vi "MegaVIEW_v_0_0_0.vi"() -> ()   [LabVIEW 2016]
panel:
  in  "Tab Control":enum32{"Setup", "Measure"}(tab)
  in  "Initalize Tempmonitor":bool
  in  "Initalize Multimeter":bool
  in  "Initalize Gaussmeter 3":bool
  in  "Initalize Gaussmeter 2":bool
  in  "Initalize Gaussmeter 1":bool
  in  "Mobile Sensor":enum32{"Sensor 1", "Sensor 2", "Sensor 3"}(radio)
  in  "Multimeter":bool
  in  "Gaussmeter 1":bool
  in  "Gaussmeter 2":bool
  in  "Gaussmeter 3":bool
  in  "Tempmonitor":bool
  in  "VISA Gaussmeter 1":refnum<visa-resource-name>
  in  "VISA Gaussmeter 2":refnum<visa-resource-name>
  in  "VISA Gaussmeter 3":refnum<visa-resource-name>
  in  "VISA Multimeter":refnum<visa-resource-name>
  in  "VISA Tempmonitor":refnum<visa-resource-name>
  in  "Method":u16(ring) items=["50 A - 50 mV Shunt", "Direct: 3 A Mode, front", "Direct: 3 A Mode, rear", "Direct: 10 A Mode"]
  in  "Type 1":u16(ring) items=["Reference (current replacement)", "Main", "Main: x-component", "Main: y-component", "Main: z-component"]
  in  "Type 2":u16(ring)
  in  "Type 3":u16(ring)
  in  "x1 [mm]":dbl
  in  "y1 [mm]":dbl
  in  "z1 [mm]":dbl
  in  "x2 [mm]":dbl
  in  "y2 [mm]":dbl
  in  "z2 [mm]":dbl
  in  "x3 [mm]":dbl
  in  "y3 [mm]":dbl
  in  "z3 [mm]":dbl
  in  "Zero Sensor 1":bool
  in  "Zero Sensor 2":bool
  in  "Zero Sensor 3":bool
  in  "Measurement Rate [Hz]":dbl
  in  "Duration [s]":dbl
  in  "Current\nReedings":dbl
  in  "Field\nReadings":dbl
  in  "Randomize Positions":bool
  in  "Position File":path
  in  "Mode":bool
  in  "hours":dbl
  in  "seconds":dbl
  in  "minutes":dbl
  in  "exit":bool
  in  "Main Graph: y-axis":u16(ring) items=["B int [mT]", "B ref [mT]", "B1 [mT]", "B2 [mT]", "B3 [mT]", "T [K]", ""]
  out "Output File":path
  out "t [s]":dbl
  out "x [mm]":dbl
  out "y [mm]":dbl
  out "z [mm]":dbl
  out "I [A]":dbl
  out "B1 [mT]":dbl
  out "B2 [mT]":dbl
  out "B3 [mT]":dbl
  out "T [K]":dbl
  in  "stop":bool
  in  "start":bool
  out "Field 1 Graph":cluster{"X":dbl, "Y":dbl}[](graph)
  out "Current Graph":cluster{"X":dbl, "Y":dbl}[](graph)
  out "Temperature Graph":cluster{"X":dbl, "Y":dbl}[](graph)
  out "Field 2 Graph":cluster{"X":dbl, "Y":dbl}[](graph)
  out "Field 3 Graph":cluster{"X":dbl, "Y":dbl}[](graph)
  out "Main Graph":cluster{"X":dbl, "Y":dbl}[](graph)
  in  "Main Graph: x-axis":u16(ring) items=["t [s]", "x [mm]", "y [mm]", "z [mm]", "I [A]", "B ref. [mT]", "B1 [mT]", "B2 [mT]", "B3 [mT]", "T [K]"]
  # "Timed"
  # "Map"
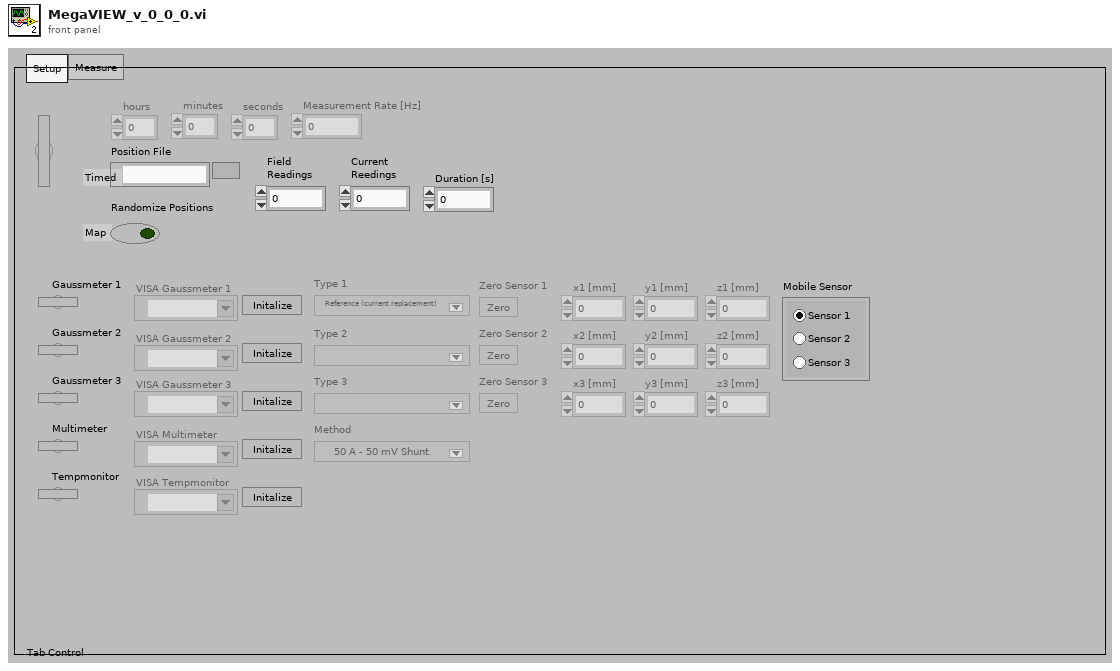
[diagram p1: front panel]
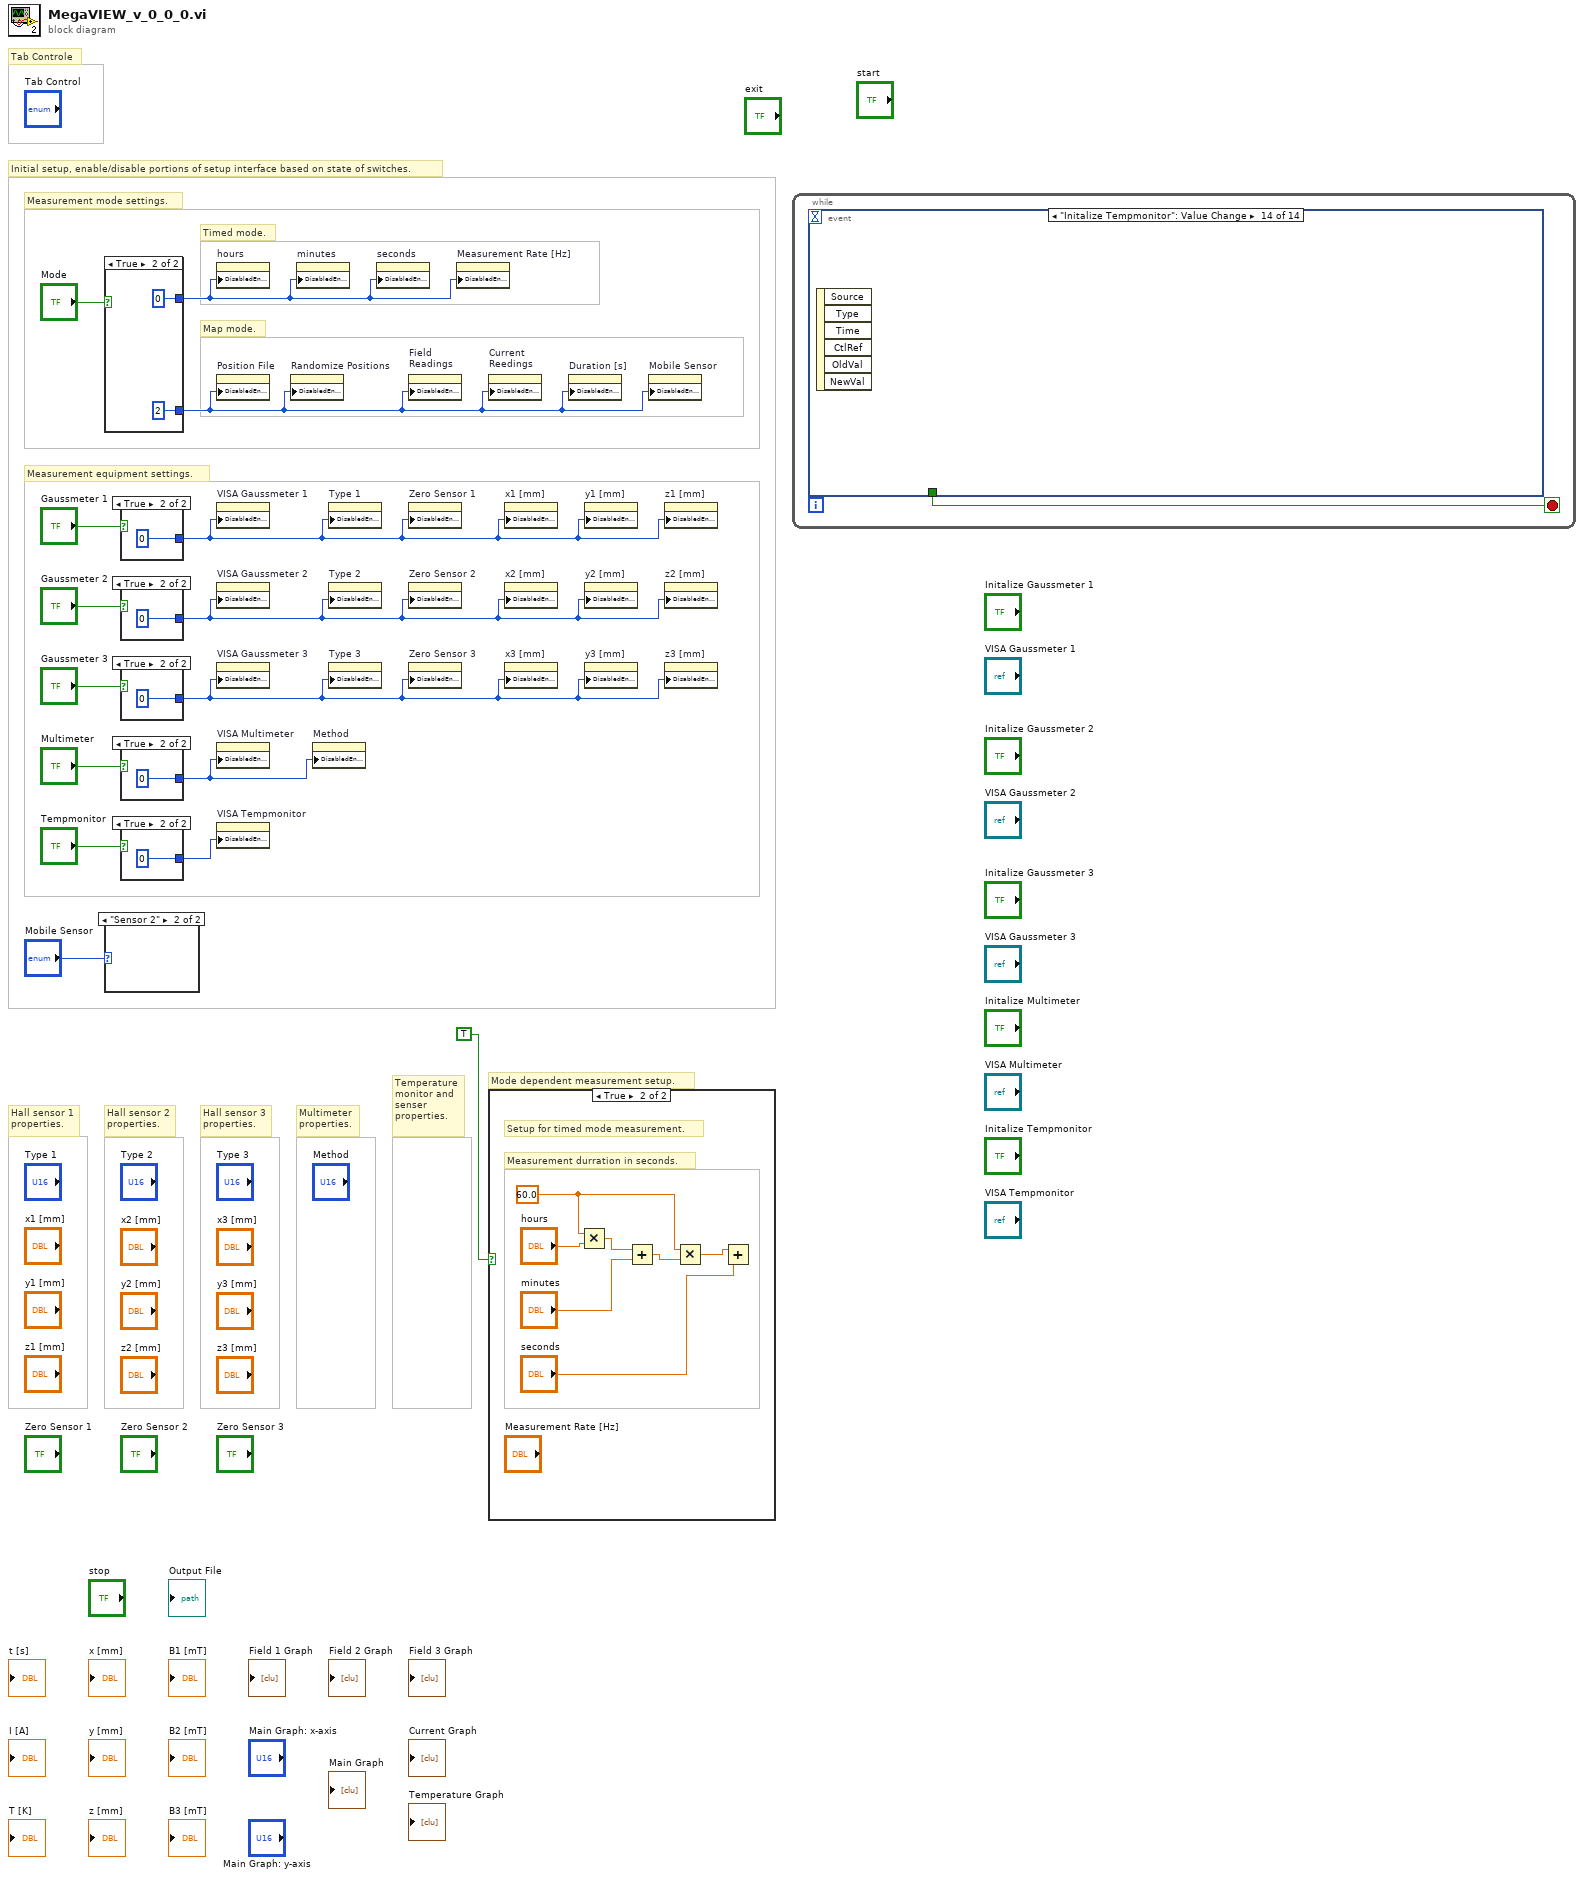
[diagram p0: block diagram]
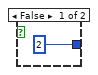
[diagram p2: hidden frame]
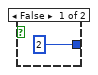
[diagram p3: hidden frame]
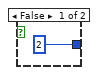
[diagram p4: hidden frame]
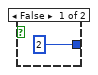
[diagram p5: hidden frame]
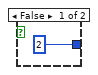
[diagram p6: hidden frame]
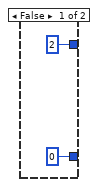
[diagram p7: hidden frame]
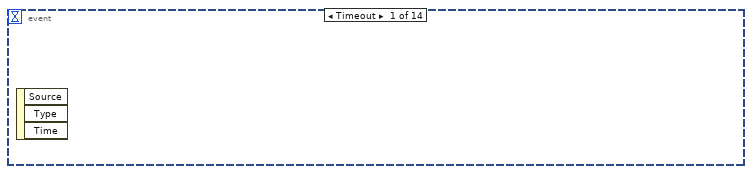
[diagram p8: hidden frame]
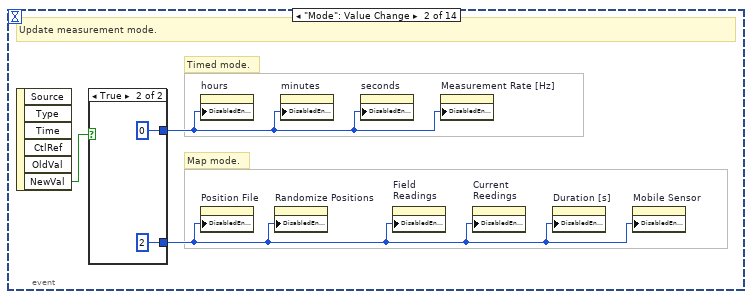
[diagram p9: hidden frame]
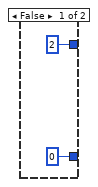
[diagram p10: hidden frame]
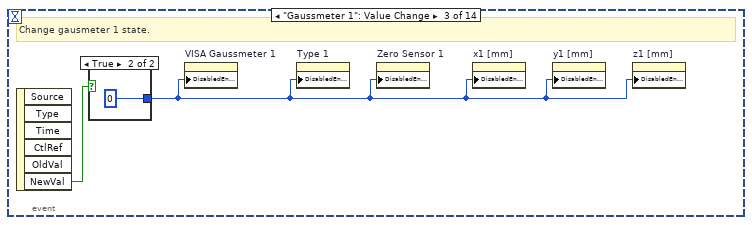
[diagram p11: hidden frame]
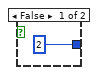
[diagram p12: hidden frame]
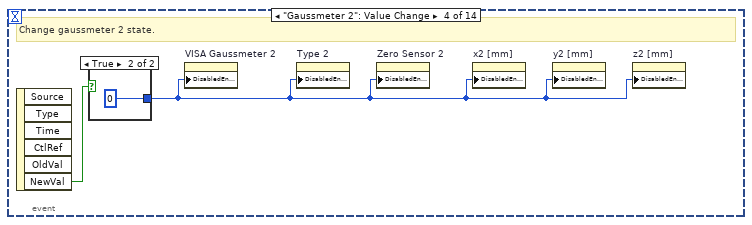
[diagram p13: hidden frame]
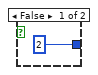
[diagram p14: hidden frame]
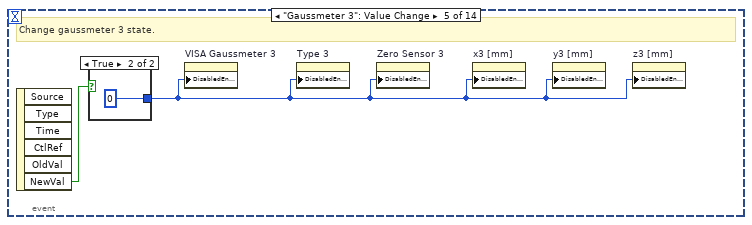
[diagram p15: hidden frame]
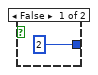
[diagram p16: hidden frame]
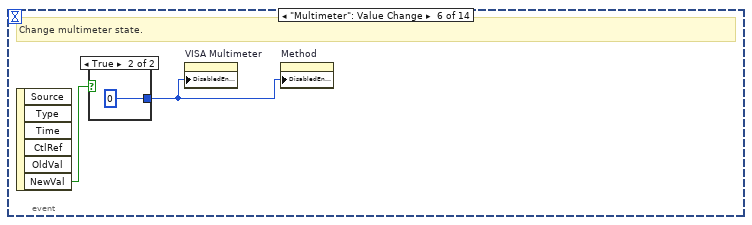
[diagram p17: hidden frame]
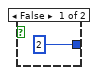
[diagram p18: hidden frame]
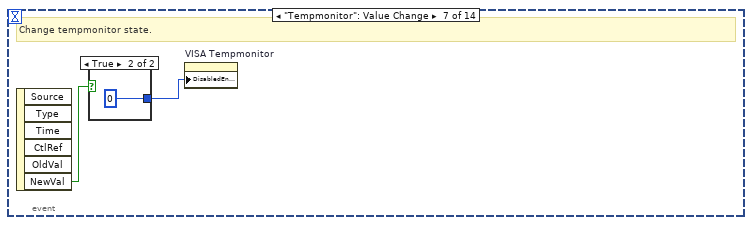
[diagram p19: hidden frame]
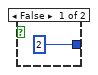
[diagram p20: hidden frame]
diagram:
  # "Measurement mode settings."
  # "Map mode."
  # "Timed mode."
  # "Temperature\nmonitor and\nsenser\nproperties."
  # "Multimeter\nproperties."
  # "Hall sensor 3\nproperties."
  # "Hall sensor 2\nproperties."
  # "Hall sensor 1\nproperties."
  # "Mode dependent measurement setup."
  # "Measurement equipment settings."
  # "Initial setup, enable/disable portions of setup interface based on state of switches."
  # "Tab Controle"
  n1 = case shown="True" "Mode" {
    tunnel: [2 i8 0] -> w12
    tunnel: [0 2] -> w13
    frame False {
    }
    frame True {
    }
  }
  n2 = case shown="\"Sensor 2\"" "Mobile Sensor" {
    frame "Sensor 1", Default {
    }
    frame "Sensor 2" {
    }
  }
  n3 = case shown="True" "Gaussmeter 1" {
    tunnel: [2 0] -> w10
    frame False {
    }
    frame True {
    }
  }
  n4 = case shown="True" "Gaussmeter 2" {
    tunnel: [2 0] -> w8
    frame False {
    }
    frame True {
    }
  }
  n5 = case shown="True" "Gaussmeter 3" {
    tunnel: [2 0] -> w6
    frame False {
    }
    frame True {
    }
  }
  n6 = case shown="True" "Multimeter" {
    tunnel: [2 0] -> w4
    frame False {
    }
    frame True {
    }
  }
  n7 = case shown="True" "Tempmonitor" {
    tunnel: [2 0] -> w2
    frame False {
    }
    frame True {
    }
  }
  n8 = property on="hours" class="DigNum (strict)"("DisabledEnum"=w12) -> ()  [unwired: 2 in, 2 out]
  n9 = property on="Position File" class="Path"("DisabledEnum"=w13) -> ()  [unwired: 2 in, 2 out]
  n10 = property on="VISA Gaussmeter 1" class="VISAName"("DisabledEnum"=w10) -> ()  [unwired: 2 in, 2 out]
  n11 = property on="VISA Gaussmeter 2" class="VISAName"("DisabledEnum"=w8) -> ()  [unwired: 2 in, 2 out]
  n12 = property on="VISA Gaussmeter 3" class="VISAName"("DisabledEnum"=w6) -> ()  [unwired: 2 in, 2 out]
  n13 = property on="VISA Multimeter" class="VISAName"("DisabledEnum"=w4) -> ()  [unwired: 2 in, 2 out]
  n14 = property on="VISA Tempmonitor" class="VISAName"("DisabledEnum"=w2) -> ()  [unwired: 2 in, 2 out]
  n15 = property on="Randomize Positions" class="Bool (strict)"("DisabledEnum"=w13) -> ()  [unwired: 2 in, 2 out]
  n16 = property on="minutes" class="DigNum (strict)"("DisabledEnum"=w12) -> ()  [unwired: 2 in, 2 out]
  n17 = property on="Method" class="Ring (strict)"("DisabledEnum"=w4) -> ()  [unwired: 2 in, 2 out]
  n18 = property on="Type 1" class="Ring (strict)"("DisabledEnum"=w10) -> ()  [unwired: 2 in, 2 out]
  n19 = property on="Type 2" class="Ring (strict)"("DisabledEnum"=w8) -> ()  [unwired: 2 in, 2 out]
  n20 = property on="Type 3" class="Ring (strict)"("DisabledEnum"=w6) -> ()  [unwired: 2 in, 2 out]
  n21 = property on="seconds" class="DigNum (strict)"("DisabledEnum"=w12) -> ()  [unwired: 2 in, 2 out]
  n22 = property on="Field\nReadings" class="DigNum (strict)"("DisabledEnum"=w13) -> ()  [unwired: 2 in, 2 out]
  n23 = property on="Zero Sensor 1" class="Bool"("DisabledEnum"=w10) -> ()  [unwired: 2 in, 2 out]
  n24 = property on="Zero Sensor 2" class="Bool"("DisabledEnum"=w8) -> ()  [unwired: 2 in, 2 out]
  n25 = property on="Zero Sensor 3" class="Bool"("DisabledEnum"=w6) -> ()  [unwired: 2 in, 2 out]
  n26 = property on="Measurement Rate [Hz]" class="DigNum (strict)"("DisabledEnum"=w12) -> ()  [unwired: 2 in, 2 out]
  n27 = property on="Current\nReedings" class="DigNum (strict)"("DisabledEnum"=w13) -> ()  [unwired: 2 in, 2 out]
  n28 = case shown="True" TRUE {
    frame False {
      # "Setup for timed mode measurement."
      n29 = Divide(x="Field\nReadings", y="Duration [s]") -> ()  [unwired: 1 out]
      n30 = Divide(x="Current\nReedings", y="Duration [s]") -> ()  [unwired: 1 out]
    }
    frame True {
      w35 = 60.0
      # "Setup for timed mode measurement."
      # "Measurement durration in seconds."
      n31 = Multiply(x=w35, y="hours") -> (x*y=w33:dbl)
      n32 = Add(x=w33, y="minutes") -> (x+y=w34:dbl)
      n33 = Multiply(x=w35, y=w34) -> (x*y=w36:dbl)
      n34 = Add(x=w36, y="seconds") -> ()  [unwired: 1 out]
    }
  }
  n35 = property on="x1 [mm]" class="DigNum (strict)"("DisabledEnum"=w10) -> ()  [unwired: 2 in, 2 out]
  n36 = property on="x2 [mm]" class="DigNum (strict)"("DisabledEnum"=w8) -> ()  [unwired: 2 in, 2 out]
  n37 = property on="x3 [mm]" class="DigNum (strict)"("DisabledEnum"=w6) -> ()  [unwired: 2 in, 2 out]
  n38 = property on="Duration [s]" class="DigNum (strict)"("DisabledEnum"=w13) -> ()  [unwired: 2 in, 2 out]
  n39 = property on="y1 [mm]" class="DigNum (strict)"("DisabledEnum"=w10) -> ()  [unwired: 2 in, 2 out]
  n40 = property on="y2 [mm]" class="DigNum (strict)"("DisabledEnum"=w8) -> ()  [unwired: 2 in, 2 out]
  n41 = property on="y3 [mm]" class="DigNum (strict)"("DisabledEnum"=w6) -> ()  [unwired: 2 in, 2 out]
  n42 = property on="Mobile Sensor" class="RadioBtnsControl (strict)"("DisabledEnum"=w13) -> ()  [unwired: 2 in, 2 out]
  n43 = property on="z1 [mm]" class="DigNum (strict)"("DisabledEnum"=w10) -> ()  [unwired: 2 in, 2 out]
  n44 = property on="z2 [mm]" class="DigNum (strict)"("DisabledEnum"=w8) -> ()  [unwired: 2 in, 2 out]
  n45 = property on="z3 [mm]" class="DigNum (strict)"("DisabledEnum"=w6) -> ()  [unwired: 2 in, 2 out]
  n46 = while {
    stop <- w40 stop-if-true
    n47 = event shown="[13] \"Initalize Tempmonitor\": Value Change" {
      selector: _ -> [_ _ _ _ _ _ _ _ _ _ _ _ _ _]
      dyn-events: _ -> [_ _ _ _ _ _ _ _ _ _ _ _ _ _]
      timeout: _ -> [_ _ _ _ _ _ _ _ _ _ _ _ _ _]
      tunnel: [_ _ _ _ _ _ _ w68 w69 _ _ _ _ _] -> w40
      event Timeout {
        n48 = event-data() -> ()  [unwired: 1 in, 3 out]
      }
      event "Mode": Value Change {
        # "Map mode."
        # "Timed mode."
        # "Update measurement mode."
        n49 = event-data() -> ("NewVal"=w41:bool)  [unwired: 1 in, 5 out]
        n50 = case shown="True" w41 {
          tunnel: [2 i8 0] -> w43
          tunnel: [0 2] -> w42
          frame False {
          }
          frame True {
          }
        }
        n51 = property on="hours" class="DigNum (strict)"("DisabledEnum"=w43) -> ()  [unwired: 2 in, 2 out]
        n52 = property on="Position File" class="Path"("DisabledEnum"=w42) -> ()  [unwired: 2 in, 2 out]
        n53 = property on="Randomize Positions" class="Bool (strict)"("DisabledEnum"=w42) -> ()  [unwired: 2 in, 2 out]
        n54 = property on="minutes" class="DigNum (strict)"("DisabledEnum"=w43) -> ()  [unwired: 2 in, 2 out]
        n55 = property on="seconds" class="DigNum (strict)"("DisabledEnum"=w43) -> ()  [unwired: 2 in, 2 out]
        n56 = property on="Field\nReadings" class="DigNum (strict)"("DisabledEnum"=w42) -> ()  [unwired: 2 in, 2 out]
        n57 = property on="Measurement Rate [Hz]" class="DigNum (strict)"("DisabledEnum"=w43) -> ()  [unwired: 2 in, 2 out]
        n58 = property on="Current\nReedings" class="DigNum (strict)"("DisabledEnum"=w42) -> ()  [unwired: 2 in, 2 out]
        n59 = property on="Duration [s]" class="DigNum (strict)"("DisabledEnum"=w42) -> ()  [unwired: 2 in, 2 out]
        n60 = property on="Mobile Sensor" class="RadioBtnsControl (strict)"("DisabledEnum"=w42) -> ()  [unwired: 2 in, 2 out]
      }
      event "Gaussmeter 1": Value Change {
        # "Change gausmeter 1 state."
        n61 = event-data() -> ("NewVal"=w48:bool)  [unwired: 1 in, 5 out]
        n62 = case shown="True" w48 {
          tunnel: [2 0] -> w49
          frame False {
          }
          frame True {
          }
        }
        n63 = property on="VISA Gaussmeter 1" class="VISAName"("DisabledEnum"=w49) -> ()  [unwired: 2 in, 2 out]
        n64 = property on="Type 1" class="Ring (strict)"("DisabledEnum"=w49) -> ()  [unwired: 2 in, 2 out]
        n65 = property on="Zero Sensor 1" class="Bool"("DisabledEnum"=w49) -> ()  [unwired: 2 in, 2 out]
        n66 = property on="x1 [mm]" class="DigNum (strict)"("DisabledEnum"=w49) -> ()  [unwired: 2 in, 2 out]
        n67 = property on="y1 [mm]" class="DigNum (strict)"("DisabledEnum"=w49) -> ()  [unwired: 2 in, 2 out]
        n68 = property on="z1 [mm]" class="DigNum (strict)"("DisabledEnum"=w49) -> ()  [unwired: 2 in, 2 out]
      }
      event "Gaussmeter 2": Value Change {
        # "Change gaussmeter 2 state."
        n69 = event-data() -> ("NewVal"=w52:bool)  [unwired: 1 in, 5 out]
        n70 = case shown="True" w52 {
          tunnel: [2 0] -> w53
          frame False {
          }
          frame True {
          }
        }
        n71 = property on="VISA Gaussmeter 2" class="VISAName"("DisabledEnum"=w53) -> ()  [unwired: 2 in, 2 out]
        n72 = property on="Type 2" class="Ring (strict)"("DisabledEnum"=w53) -> ()  [unwired: 2 in, 2 out]
        n73 = property on="Zero Sensor 2" class="Bool"("DisabledEnum"=w53) -> ()  [unwired: 2 in, 2 out]
        n74 = property on="x2 [mm]" class="DigNum (strict)"("DisabledEnum"=w53) -> ()  [unwired: 2 in, 2 out]
        n75 = property on="y2 [mm]" class="DigNum (strict)"("DisabledEnum"=w53) -> ()  [unwired: 2 in, 2 out]
        n76 = property on="z2 [mm]" class="DigNum (strict)"("DisabledEnum"=w53) -> ()  [unwired: 2 in, 2 out]
      }
      event "Gaussmeter 3": Value Change {
        # "Change gaussmeter 3 state."
        n77 = event-data() -> ("NewVal"=w56:bool)  [unwired: 1 in, 5 out]
        n78 = case shown="True" w56 {
          tunnel: [2 0] -> w57
          frame False {
          }
          frame True {
          }
        }
        n79 = property on="VISA Gaussmeter 3" class="VISAName"("DisabledEnum"=w57) -> ()  [unwired: 2 in, 2 out]
        n80 = property on="Type 3" class="Ring (strict)"("DisabledEnum"=w57) -> ()  [unwired: 2 in, 2 out]
        n81 = property on="Zero Sensor 3" class="Bool"("DisabledEnum"=w57) -> ()  [unwired: 2 in, 2 out]
        n82 = property on="x3 [mm]" class="DigNum (strict)"("DisabledEnum"=w57) -> ()  [unwired: 2 in, 2 out]
        n83 = property on="y3 [mm]" class="DigNum (strict)"("DisabledEnum"=w57) -> ()  [unwired: 2 in, 2 out]
        n84 = property on="z3 [mm]" class="DigNum (strict)"("DisabledEnum"=w57) -> ()  [unwired: 2 in, 2 out]
      }
      event "Multimeter": Value Change {
        # "Change multimeter state."
        n85 = event-data() -> ("NewVal"=w60:bool)  [unwired: 1 in, 5 out]
        n86 = case shown="True" w60 {
          tunnel: [2 0] -> w61
          frame False {
          }
          frame True {
          }
        }
        n87 = property on="VISA Multimeter" class="VISAName"("DisabledEnum"=w61) -> ()  [unwired: 2 in, 2 out]
        n88 = property on="Method" class="Ring (strict)"("DisabledEnum"=w61) -> ()  [unwired: 2 in, 2 out]
      }
      event "Tempmonitor": Value Change {
        # "Change tempmonitor state."
        n89 = event-data() -> ("NewVal"=w64:bool)  [unwired: 1 in, 5 out]
        n90 = case shown="True" w64 {
          tunnel: [2 0] -> w65
          frame False {
          }
          frame True {
          }
        }
        n91 = property on="VISA Tempmonitor" class="VISAName"("DisabledEnum"=w65) -> ()  [unwired: 2 in, 2 out]
      }
      event "start": Value Change {
        # "Start measurement."
        n92 = event-data() -> ("NewVal"=w68:bool)  [unwired: 1 in, 5 out]
      }
      event "exit": Value Change {
        n93 = event-data() -> ("NewVal"=w69:bool)  [unwired: 1 in, 5 out]
      }
      event "Initalize Gaussmeter 1": Value Change {
        n94 = event-data() -> ()  [unwired: 1 in, 6 out]
      }
      event "Initalize Gaussmeter 2": Value Change {
        n95 = event-data() -> ()  [unwired: 1 in, 6 out]
      }
      event "Initalize Gaussmeter 3": Value Change {
        n96 = event-data() -> ()  [unwired: 1 in, 6 out]
      }
      event "Initalize Multimeter": Value Change {
        n97 = event-data() -> ()  [unwired: 1 in, 6 out]
      }
      event "Initalize Tempmonitor": Value Change {
        n98 = event-data() -> ()  [unwired: 1 in, 6 out]
      }
    }
  }
